vi "GetTimeout.vi"(8 "error in (no error)":errorcluster, 11 "Ticker In":refnum<class "Ticker.lvclass">) -> (0 "error out":errorcluster, 1 "Time left":i32, 2 "timed out":bool, 3 "Ticker Out":refnum<class "Ticker.lvclass">)   [LabVIEW 2025, in "Ticker.lvclass"]
uses:
  Ticker.lvclass
  Ticker.lvclass/Ticker.ctl
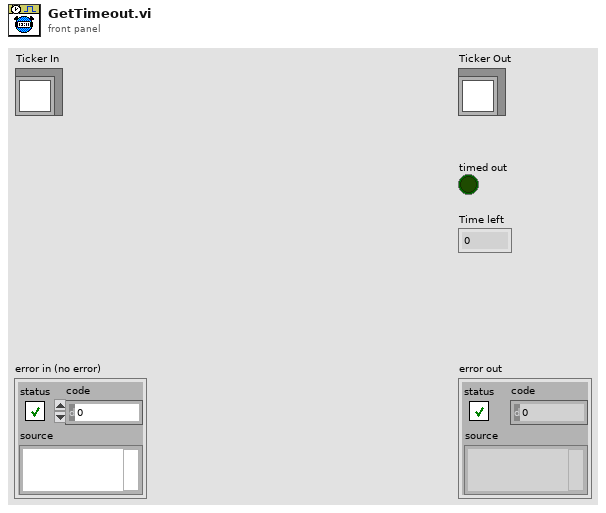
[diagram p1: front panel]
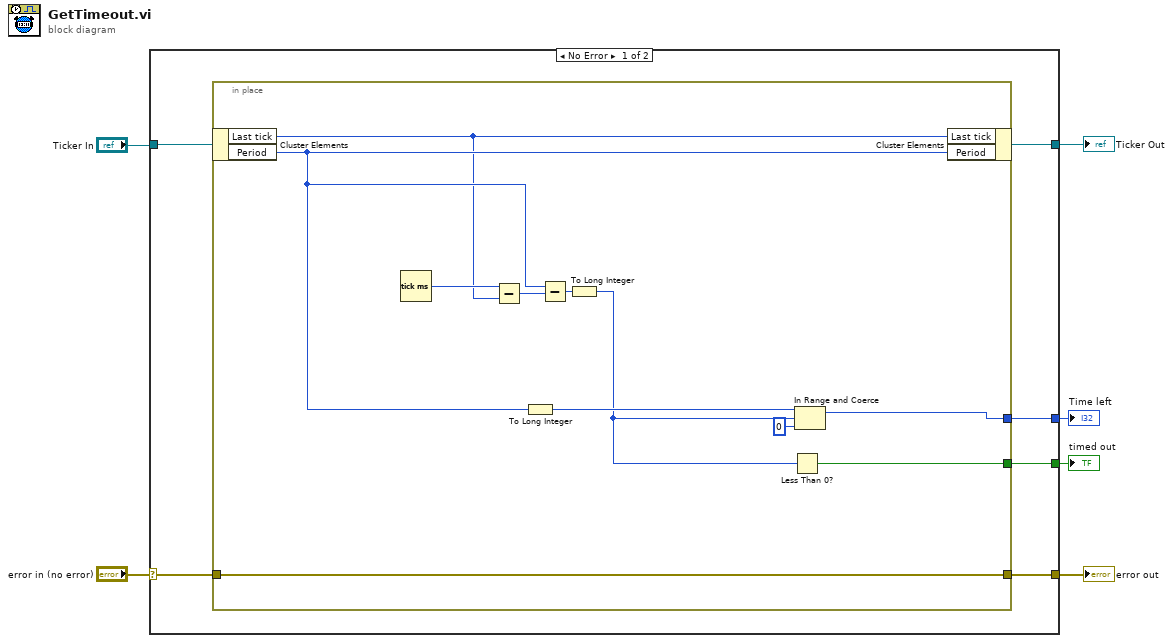
[diagram p0: block diagram]
diagram:
  n1 = case shown="No Error" "error in (no error)" {
    selector: "error in (no error)" -> [w9 w25]
    tunnel: [w10 w25] -> w4
    tunnel: [w11 w24] -> w5
    tunnel: "Ticker In" -> [w12 w24]
    tunnel: [w8 _] -> w2
    tunnel: [w7 _] -> w1
    frame No Error {
      n2 = in-place {
        in-place-border: [w23] -> w10
        in-place-border: w9 -> [w23]
        in-place-border: [w15] -> w8
        in-place-border: [w13] -> w7
        n3 = in-place-cluster #1(w12) -> ("Last tick"=w16:u32, "Period"=w17:u32)
        n4 = Tick Count (ms)() -> (millisecond timer value=w20:u32)
        n5 = Subtract(x=w20, y=w16) -> (x-y=w22:u32)
        n6 = To Long Integer(number=w17) -> (32bit integer=w18:i32)
        n7 = Subtract(x=w17, y=w22) -> (x-y=w21:u32)
        n8 = To Long Integer(number=w21) -> (32bit integer=w14:i32)
        n9 = Less Than 0?(x=w14) -> (x < 0?=w13:bool)
        n10 = In Range and Coerce(upper limit=w18, x=w14, lower limit=0) -> (coerced(x)=w15:i32)  [unwired: 1 out]
        n11 = in-place-cluster #1("Last tick"=w16, "Period"=w17) -> (w11:refnum<class "Ticker.lvclass">)
      }
    }
    frame Error {
    }
  }
  "error out" <- w4
  "Ticker Out" <- w5
  "Time left" <- w2
  "timed out" <- w1
